vi "GPS Loop.vi"() -> ()   [LabVIEW 2009]
uses:
  TypeDefs/Sensor Typedefs/GPS Data.ctl
  <vilib>/Instr/_visa.llb/VISA Configure Serial Port (Instr).vi
  <vilib>/Platform/TimedLoop/XDataNode/XDataNode.xnode
  <vilib>/Platform/TimedLoop/XDataNode/loadlvalarms.vi
  <vilib>/Platform/TimedLoop/XDataNode/timing_clust.ctl
  <vilib>/Platform/TimedLoop/XDataNode/nitl_modes.ctl
  <vilib>/Platform/TimedLoop/XDataNode/wakeup.ctl
  UDP Lib/UDP Network Location.ctl
  <vilib>/Platform/TimedLoop/XDataNode/XDNodeRunTimeDep.lvlib
  <vilib>/NI_Real-Time Target Support.lvlib
panel:
  out "error out":errorcluster
  out "Output Started":bool
  out "Output Halted":bool
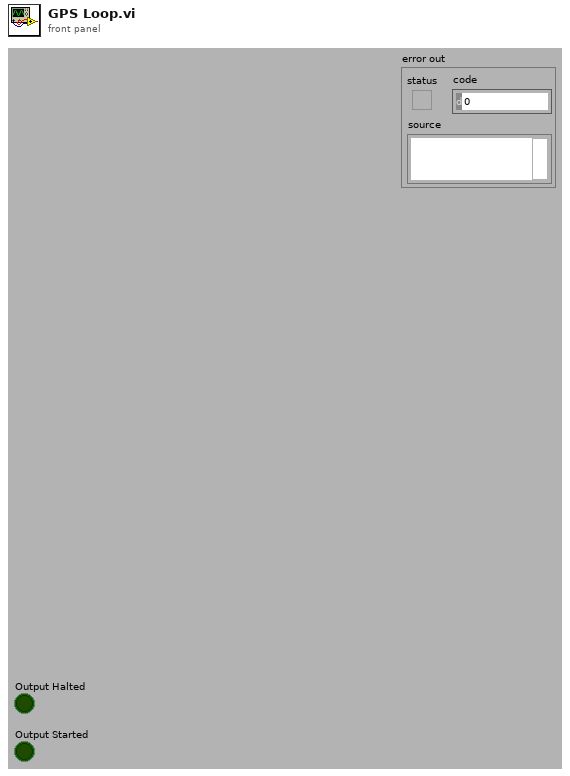
[diagram p1: front panel]
types:
  T1 = typedef "GPS Data.ctl" = cluster{"Latitude":dbl, "Longitude":dbl}
  T2 = typedef "UDP Base.ctl" = cluster{"UDP Session":refnum<k16>, "UDP Socket Params":T3}
  T3 = typedef "UDP Socket Params.ctl" = cluster{"Local Port":u16, "Read Timeout":i32, "Write Timeout":i32}
  T4 = typedef "XDNodeRunTimeDep.lvlib/timing_clust.ctl" = cluster{"Expected End [f-1]":u64, "Actual End [f-1]":u64, "Finished Late? [f-1]":bool, "Expected End [i-1]":u64, "Actual End [i-1]":u64, "Finished Late? [i-1]":bool, "Expected Start [i]":u64, "Actual Start [i]":u64, "Expected Start [f]":u64, "Actual Start [f]":u64, "Source Name":string, "Structure Name":string, "Period":i64, "Deadline":i64, "Offset":i64, "Start":i64, "Priority":i32, "Timeout":i32, "Mode":T5, "Wakeup Reason":T6, "Error":errorcluster, "Source Type":string, "Secondary Source Type":string, "Global End Time":u64, "Global Start Time":u64, "Frame Duration":u64, "Iteration Duration":u64, "Assigned CPU":i32, "I/O Scan Engine Mode":u32}
  T5 = typedef "XDNodeRunTimeDep.lvlib/nitl_modes.ctl" = enum32{"No Change", "Process missed periods, maintain original phase", "Discard missed periods, maintain original phase", "Process missed periods, ignore original phase", "Discard missed periods, ignore original phase"}
  T6 = typedef "XDNodeRunTimeDep.lvlib/wakeup.ctl" = enum32{"Normal", "Aborted", "Asynchronous wakeup", "Timing source error", "Timed loop error", "Timeout"}
  T7 = typedef "UDP Network Location.ctl" = cluster{"IP Address":string, "Port":u16}
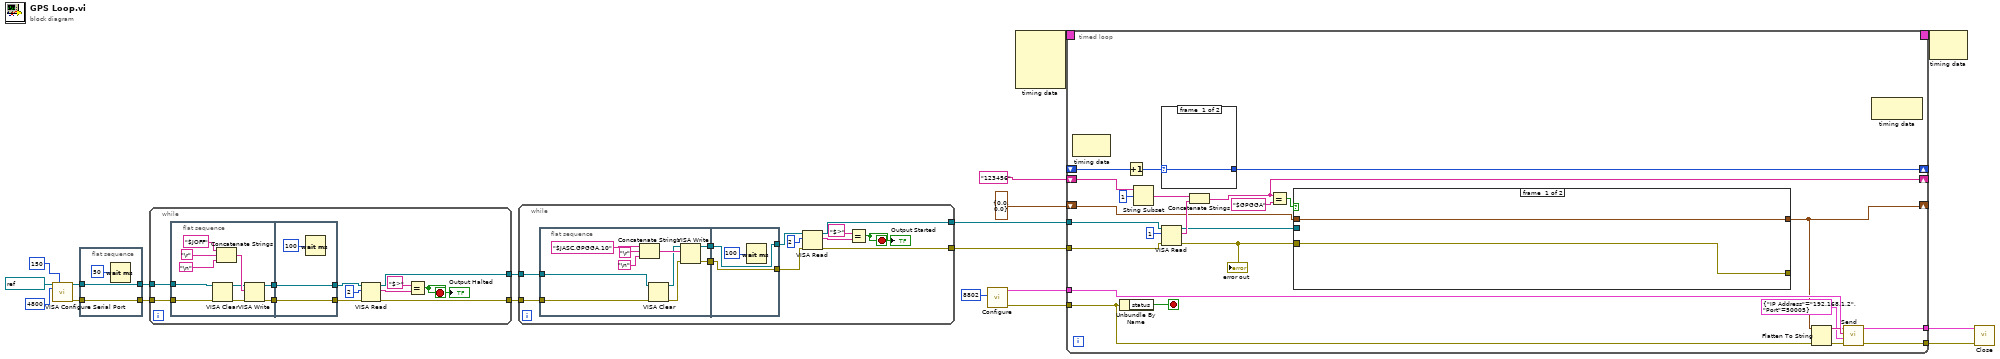
[diagram p0: block diagram]
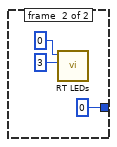
[diagram p2: hidden frame]
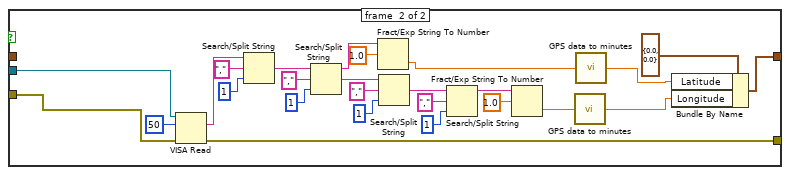
[diagram p3: hidden frame]
diagram:
  n1 = call-poly "VISA Configure Serial Port"("VISA resource name"=refnum<visa-resource-name> "COM1", "timeout (10sec)"=u32 150, "baud rate (9600)"=u32 4800) -> ("VISA resource name out"=w7:refnum<visa-resource-name>, "error out"=w9:errorcluster)  [unwired: 11 in]
  n2 = flat-sequence {
    tunnel: [w21] -> w6
    tunnel: w9 -> [w21]
    tunnel: w7 -> [w22]
    tunnel: [w22] -> w5
    frame #0 {
      n3 = Wait (ms)(milliseconds to wait=u32 50) -> ()  [unwired: 1 out]
    }
  }
  n4 = while {
    tunnel: w6 -> [w35]
    tunnel: w5 -> [w34]
    tunnel: [w29] -> w3
    tunnel: [w28] -> w4
    stop <- w30 stop-if-true
    n5 = flat-sequence {
      tunnel: w35 -> [w45]
      tunnel: w34 -> [w44]
      tunnel: [w39] -> w26
      tunnel: [w36] -> w24
      tunnel: [w47] -> w27
      tunnel: w26 -> [w47]
      tunnel: [w46] -> w25
      tunnel: w24 -> [w46]
      frame #0 {
        n6 = VISA Clear(VISA resource name=w44, error in (no error)=w45) -> (VISA resource name out=w37:refnum<visa-resource-name>, error out=w38:errorcluster)
        n7 = Concatenate Strings("$JOFF" ("Ascii to write 2"), "\r", "\n") -> (w42:string)
        n8 = VISA Write(VISA resource name=w37, write buffer=w42, error in (no error)=w38) -> (VISA resource name out=w36:refnum<visa-resource-name>, error out=w39:errorcluster)  [unwired: 1 out]
      }
      frame #1 {
        n9 = Wait (ms)(milliseconds to wait=u32 100) -> ()  [unwired: 1 out]
      }
    }
    n10 = VISA Read(VISA resource name=w25, byte count=u32 2, error in (no error)=w27) -> (VISA resource name out=w28:refnum<visa-resource-name>, read buffer=w32:string, error out=w29:errorcluster)  [unwired: 1 out]
    n11 = Equal?(x="$>" ("read buffer"), y=w32) -> (x = y?=w30:bool)
    "Output Halted" <- w30
  }
  n12 = while {
    tunnel: w3 -> [w60]
    tunnel: w4 -> [w59]
    tunnel: [w54] -> w1
    tunnel: [w53] -> w2
    stop <- w55 stop-if-true
    n13 = flat-sequence {
      tunnel: w60 -> [w70]
      tunnel: w59 -> [w69]
      tunnel: [w64] -> w51
      tunnel: [w61] -> w49
      tunnel: [w72] -> w52
      tunnel: w51 -> [w72]
      tunnel: [w71] -> w50
      tunnel: w49 -> [w71]
      frame #0 {
        n14 = Concatenate Strings("$JASC,GPGGA,10" ("Ascii to write 2"), "\r", "\n") -> (w67:string)
        n15 = VISA Clear(VISA resource name=w69, error in (no error)=w70) -> (VISA resource name out=w62:refnum<visa-resource-name>, error out=w63:errorcluster)
        n16 = VISA Write(VISA resource name=w62, write buffer=w67, error in (no error)=w63) -> (VISA resource name out=w61:refnum<visa-resource-name>, error out=w64:errorcluster)  [unwired: 1 out]
      }
      frame #1 {
        n17 = Wait (ms)(milliseconds to wait=u32 100) -> ()  [unwired: 1 out]
      }
    }
    n18 = VISA Read(VISA resource name=w50, byte count=u32 2, error in (no error)=w52) -> (VISA resource name out=w53:refnum<visa-resource-name>, read buffer=w57:string, error out=w54:errorcluster)  [unwired: 1 out]
    n19 = Equal?(x="$>" ("read buffer"), y=w57) -> (x = y?=w55:bool)
    "Output Started" <- w55
  }
  n20 = call "Configure.vi"("Local Port"=u16 8802) -> ("error out"=w17:errorcluster, "UDP Base out"=w18:T2)  [unwired: 9 in]
  n21 = node-c288() -> (w14:T4)  [unwired: 4 in]
  n22 = timed-loop {
    tunnel: w2 -> [w90]
    tunnel: w1 -> [w89]
    shift-right: [w87] -> _
    shift-left: "123456" -> [w88]
    shift-right: [w74] -> _
    shift-left: T1 {"Latitude"=0.0, "Longitude"=0.0} ("GPS Point") -> [w86]
    tunnel: w18 -> [w83]
    tunnel: w17 -> [w80]
    tunnel: [w82] -> w16
    tunnel: [w81] -> w15
    timing: w14 -> [_]
    timing-out: [_] -> w13
    shift-right: [w75] -> _
    shift-left: _ -> [w77]
    stop <- w79 stop-if-true
    n23 = node-c288() -> ()  [unwired: 1 in, 1 out]
    n24 = Unbundle By Name(w80) -> ("status"=w79:bool)
    n25 = Increment(x=w77) -> (x+1=w76:i32)
    n26 = String Subset(string=w88, offset (0)=1) -> (substring=w95:string)  [unwired: 1 in]
    n27 = case shown="2" w76 {
      selector: w76 -> [w99 _]
      tunnel: [w99 0] -> w75
      frame #0 {
      }
      frame #1 {
        n28 = call <vilib>:"RT LEDs.vi"("State"=3, "LED Num"=0) -> ()  [unwired: 4 in, 2 out]
      }
    }
    n29 = VISA Read(VISA resource name=w90, byte count=u32 1, error in (no error)=w89) -> (VISA resource name out=w91:refnum<visa-resource-name>, read buffer=w96:string, error out=w92:errorcluster)  [unwired: 1 out]
    "error out" <- w92
    n30 = Concatenate Strings(w95, w96) -> (w87:string)
    n31 = Equal?(x=w87, y="$GPGGA") -> (x = y?=w93:bool)
    n32 = case shown="True" w93 {
      tunnel: w91 -> [_ w112]
      tunnel: w92 -> [w106 w111]
      tunnel: [w106 w120] -> _
      tunnel: [w105 w114] -> w74
      tunnel: w86 -> [w105 _]
      frame #0 {
      }
      frame #1 {
        n33 = VISA Read(VISA resource name=w112, byte count=u32 50, error in (no error)=w111) -> (read buffer=w119:string, error out=w120:errorcluster)  [unwired: 2 out]
        n34 = Search/Split String(string=w119, search string/char (-)=",", offset (0)=1) -> (match + rest of string=w125:string)  [unwired: 2 out]
        n35 = Search/Split String(string=w125, search string/char (-)=",", offset (0)=1) -> (substring before match=w115:string, match + rest of string=w124:string)  [unwired: 1 out]
        n36 = Fract/Exp String To Number(string=w115, offset=1.0 ("default (0 DBL)")) -> (number=w110:dbl)  [unwired: 2 in, 1 out]
        n37 = Search/Split String(string=w124, search string/char (-)=",", offset (0)=1) -> (match + rest of string=w121:string)  [unwired: 2 out]
        n38 = Search/Split String(string=w121, search string/char (-)=",", offset (0)=1) -> (substring before match=w118:string)  [unwired: 2 out]
        n39 = Fract/Exp String To Number(string=w118, offset=1.0 ("default (0 I32)")) -> (number=w109:dbl)  [unwired: 2 in, 1 out]
        n40 = call "GPS data to minutes.vi"("GPS Data in (DDmm.mm)"=w109) -> ("GPS Data out (in minutes)"=w107:dbl)
        n41 = call "GPS data to minutes.vi"("GPS Data in (DDmm.mm)"=w110) -> ("GPS Data out (in minutes)"=w108:dbl)
        n42 = Bundle By Name(cluster=T1 {"Latitude"=0.0, "Longitude"=0.0} ("GPS Point"), "Latitude"=w108, "Longitude"=w107) -> (w114:T1)
      }
    }
    n43 = Flatten To String(anything=w74, error in (no error)=w80) -> (data string=w84:string, error out=w85:errorcluster)  [unwired: 2 in, 1 out]
    n44 = call "Send.vi"("error in (no error)"=w85, "Destination Location"=T7 {"IP Address"="192.168.1.2", "Port"=50005} ("cRIO Network Location"), "Send Data"=w84, "UDP Base in"=w83) -> ("error out"=w81:errorcluster, "UDP Base out"=w82:T2)  [unwired: 5 in, 1 out]
    n45 = node-c288() -> ()  [unwired: 1 in, 1 out]
  }
  n46 = node-c288(w13) -> ()  [unwired: 1 out]
  n47 = call "Close.vi"("error in (no error)"=w15, "Cluster of class private data"=w16) -> ()  [unwired: 9 in, 1 out]
